vi "HandleItemActivation.vi"(8 "error in (no error)":errorcluster, 11 "Help in":refnum<class "Help.lvclass">) -> (0 "error out":errorcluster, 3 "Help out":refnum<class "Help.lvclass">)   [LabVIEW 2009, in "NavScreen.lvlib" / "Help.lvclass"]
uses:
  Help.lvclass
  Help.lvclass/Help.ctl
  <vilib>/Platform/browser.llb/Open URL in Default Browser (string).vi
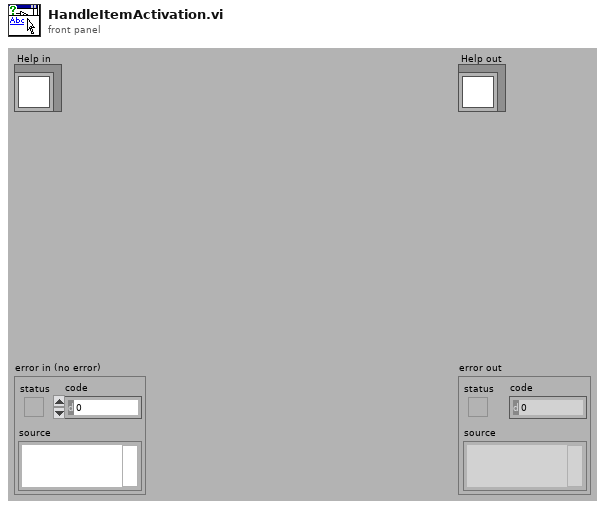
[diagram p1: front panel]
types:
  T1 = enum32{"invalid OS target", "Mac OS", "Windows 3.1", "Windows 95/NT", "Solaris 1", "Solaris 2", "HP-UX", "PowerMAX", "Linux", "Irix", "Rhapsody", "BeOS", "AIX", "OSF1", "VxWorks", "PharLap", "Carbon", "RTX", "Windows x64", "Linux x64"}
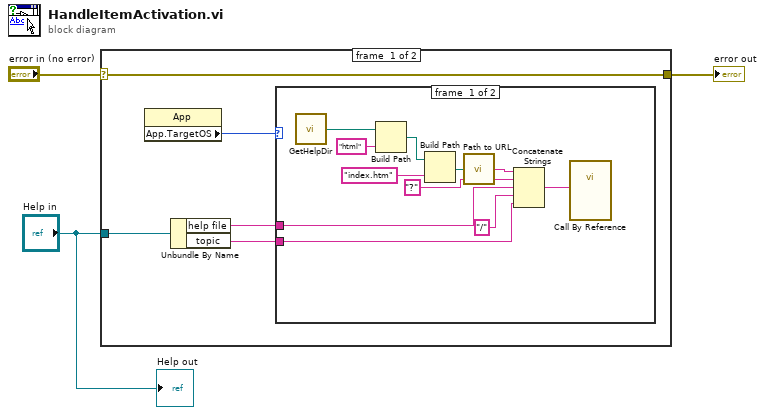
[diagram p0: block diagram]
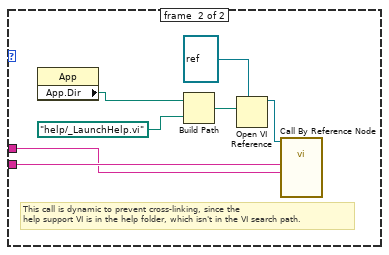
[diagram p2: hidden frame]
diagram:
  n1 = case shown="No Error" "error in (no error)" {
    selector: "error in (no error)" -> [w8 w27]
    tunnel: [w8 w27] -> w2
    tunnel: "Help in" -> [w6 _]
    frame #0 {
      n2 = property on="Property Node" class="App"() -> ("App.TargetOS"=w7:T1)  [unwired: 2 in, 2 out]
      n3 = Unbundle By Name(w6) -> ("help file"=w5:string, "topic"=w4:string)
      n4 = case shown="\"Linux\", \"Carbon\"" w7 {
        tunnel: w5 -> [w10 w20]
        tunnel: w4 -> [w15 w21]
        frame #0 {
          n5 = call <vilib>:"GetHelpDir.vi"() -> ("help path"=w14:path)
          n6 = Build Path(base path=w14, name or relative path="html") -> (appended path=w18:path)
          n7 = Build Path(base path=w18, name or relative path="index.htm") -> (appended path=w17:path)
          n8 = call <vilib>:"Path to URL.vi"("path"=w17) -> ("url"=w16:string)
          n9 = Concatenate Strings(w16, "?" ("string"), w10, "/" ("string"), w15) -> (w9:string)
          n10 = call-by-ref "?"("URL"=w9) -> ()  [unwired: 7 in, 4 out]
        }
        frame #1 {
          # "This call is dynamic to prevent cross-linking, since the\nhelp support VI is in the help folder, which isn't in the VI search path."
          n11 = property on="Property Node" class="App"() -> ("App.Dir"=w25:path)  [unwired: 2 in, 2 out]
          n12 = Build Path(base path=w25, name or relative path=path "help/_LaunchHelp.vi") -> (appended path=w24:path)
          n13 = Open VI Reference(type specifier VI Refnum (for type only)=refnum<vi> refnum, vi path=w24) -> (vi reference=w23:refnum<vi>)  [unwired: 4 in, 1 out]
          n14 = call-by-ref "Call By Reference Node"(reference=w23, "CHM or HLP filename (lvdialog.chm)"=w20, "HTML filename"=w21) -> ()  [unwired: 6 in, 3 out]
        }
      }
    }
    frame #1 {
    }
  }
  "error out" <- w2
  "Help out" <- "Help in"
